vi "Timer.vi"() -> ()   [LabVIEW 2019]
panel:
  in  "Timer":dbl
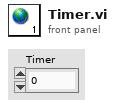
[diagram p1: front panel]
diagram:
